vi "Pull_Data_via_Public_Client.vi"(0 "Path of File relative to EnFlo Data Root":path[](array[path]), 1 "application reference":refnum<vi>, 2 "Running on Server?":bool, 3 "Archive Files?":bool, 5 "error in (no error)":errorcluster) -> (6 "Error String":string, 7 "Problem Files":path[](array[path]), 8 "error out":errorcluster)   [LabVIEW 2018]
uses:
  Anemometry/Anemometry Sub Vis/Globals/Constants_global.vi
  Sub VIs/Harvest_Global.vi
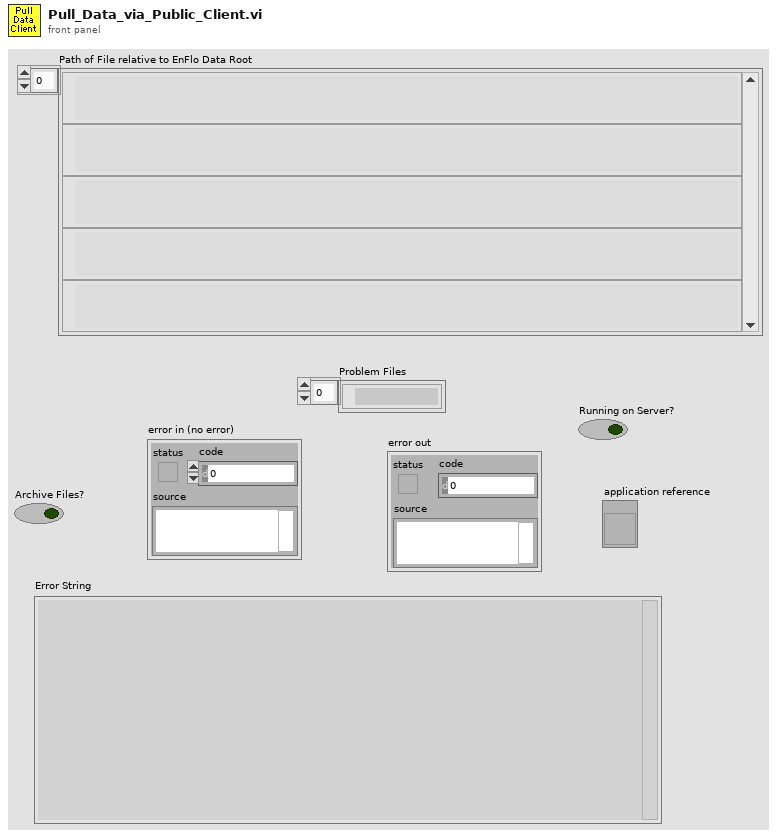
[diagram p1: front panel]
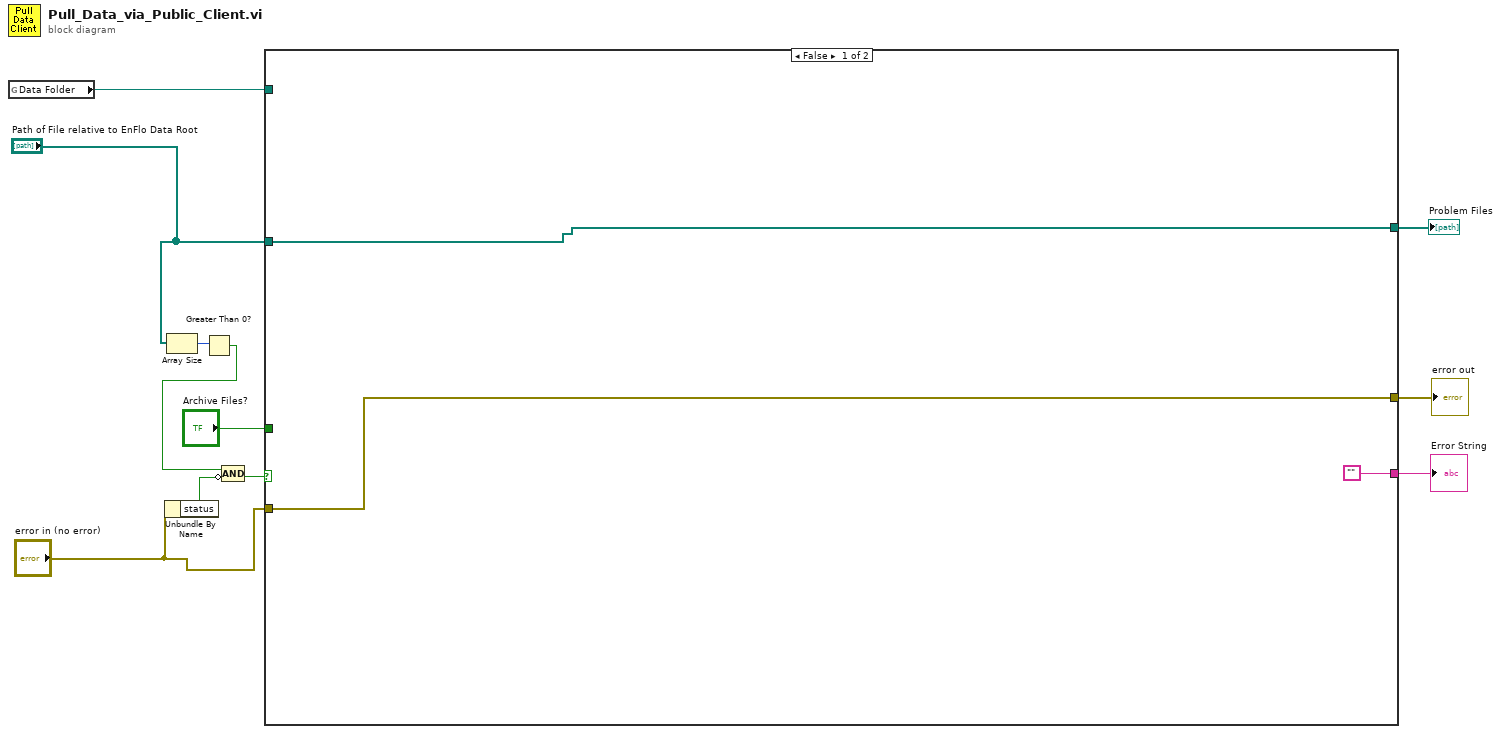
[diagram p0: block diagram]
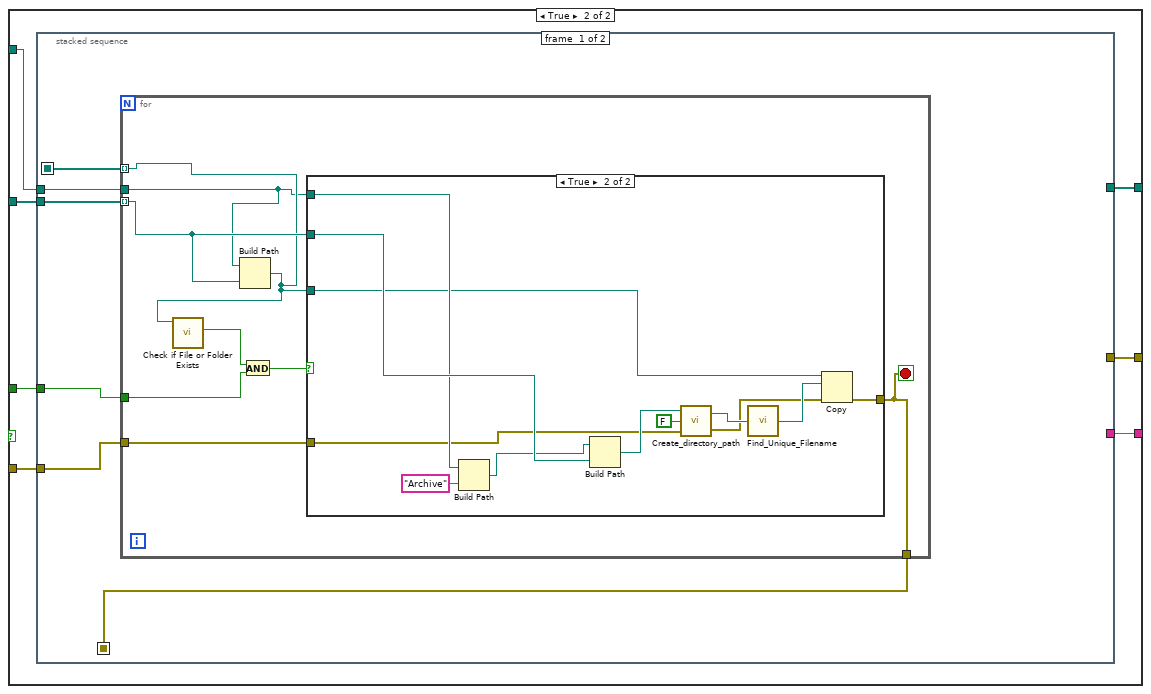
[diagram p2: hidden frame]
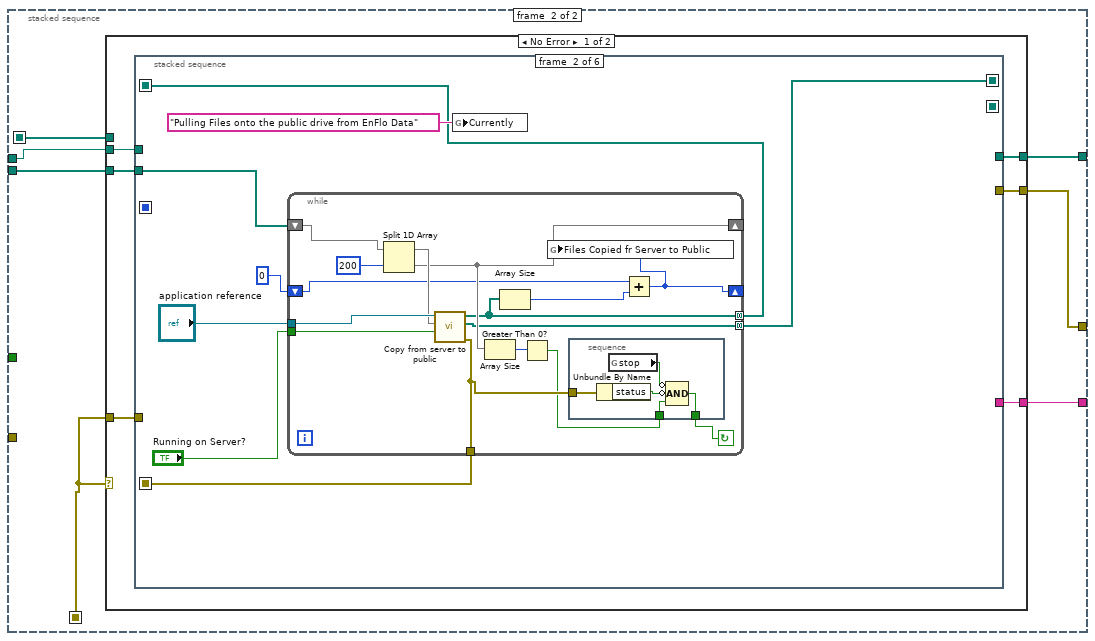
[diagram p4: hidden frame]
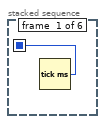
[diagram p5: hidden frame]
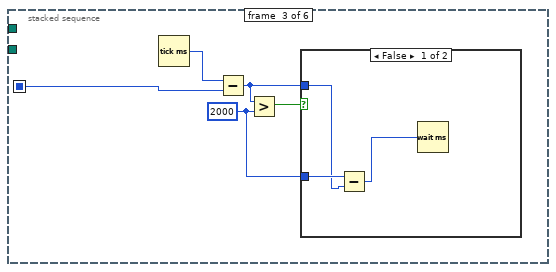
[diagram p6: hidden frame]
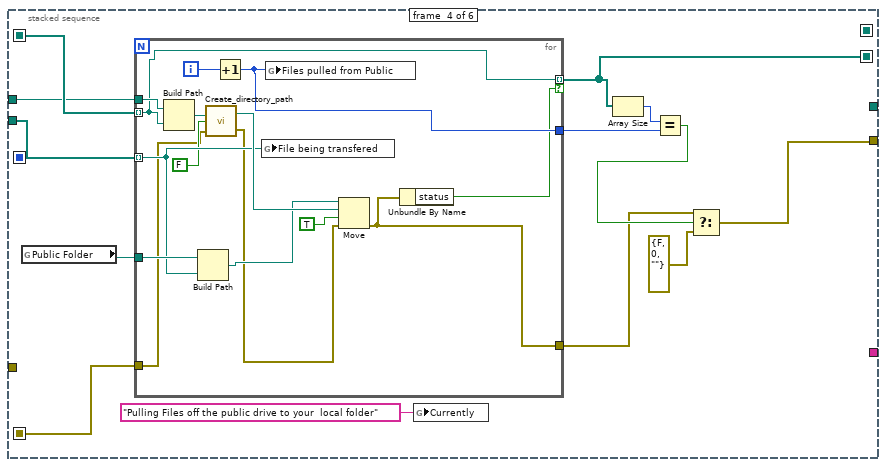
[diagram p8: hidden frame]
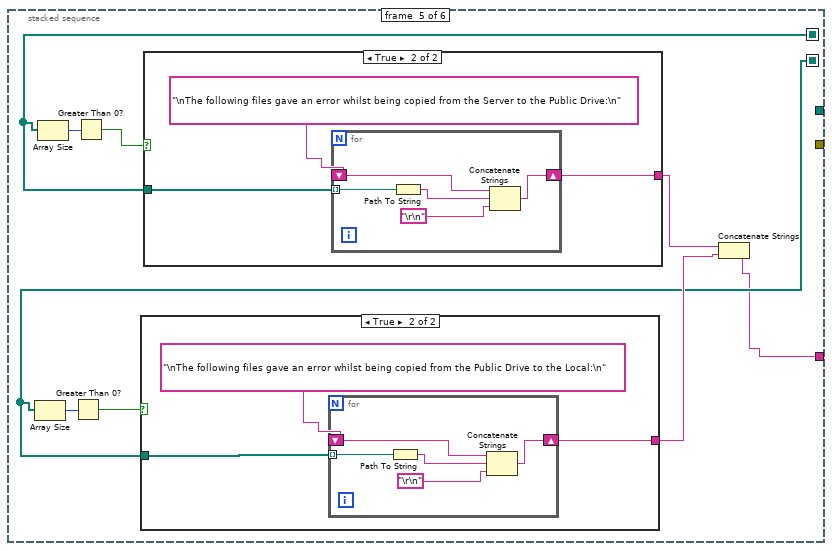
[diagram p9: hidden frame]
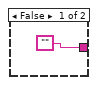
[diagram p10: hidden frame]
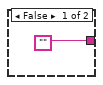
[diagram p11: hidden frame]
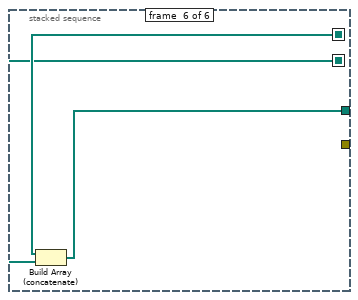
[diagram p12: hidden frame]
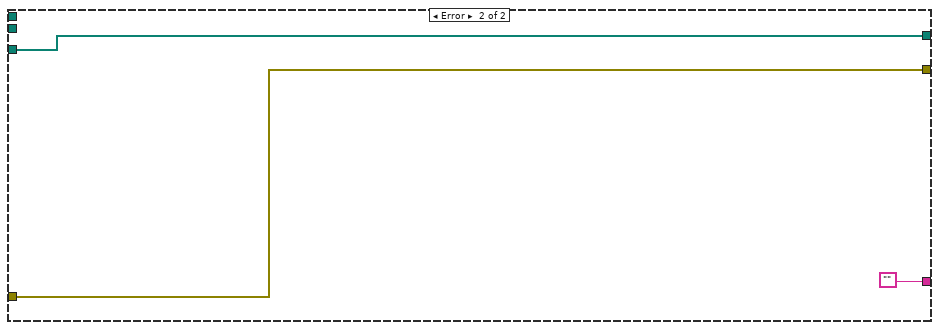
[diagram p13: hidden frame]
diagram:
  n1 = global read "Constants_global.vi" "Data Folder"() -> (w9:path)
  n2 = Unbundle By Name("error in (no error)") -> ("status"=w8:bool)
  n3 = Array Size(array="Path of File relative to EnFlo Data Root") -> (size(s)=w7:i32)
  n4 = Greater Than 0?(x=w7) -> (x > 0?=w6:bool)
  n5 = Compound Arithmetic op=AND(w6, invert w8) -> (w4:bool)
  n6 = case shown="False" w4 {
    tunnel: [w14 w21] -> w11
    tunnel: "error in (no error)" -> [w14 w20]
    tunnel: "Path of File relative to EnFlo Data Root" -> [w12 w19]
    tunnel: "Archive Files?" -> [_ w18]
    tunnel: w9 -> [_ w17]
    tunnel: ["" w16] -> w2
    tunnel: [w12 w15] -> w1
    frame False {
    }
    frame True {
      n7 = stacked-sequence {
        seq-local: [w26 _] -> [_ w52]
        seq-local: [w24 _] -> [_ w54]
        tunnel: [_ w55] -> w21
        tunnel: w20 -> [w27 _]
        tunnel: w19 -> [w25 w53]
        tunnel: w18 -> [w23 _]
        tunnel: w17 -> [w22 w51]
        tunnel: [_ w50] -> w16
        tunnel: [_ w49] -> w15
        frame #0 {
          n8 = for {
            tunnel: w27 -> [w35]
            tunnel: [w30] -> w26
            tunnel: w25 -> [w34] mode=indexing
            tunnel: w23 -> [w33]
            tunnel: [w29] -> w24 mode=indexing
            tunnel: w22 -> [w28]
            stop <- w30 stop-if-true
            n9 = Build Path(base path=w28, name or relative path=w34) -> (appended path=w29:path)
            n10 = call <vilib>:"Check if File or Folder Exists.vi"("path"=w29) -> ("file or folder exists?"=w32:bool)  [unwired: 8 in, 2 out]
            n11 = And(x=w32, y=w33) -> (x .and. y?=w31:bool)
            n12 = case shown="True" w31 {
              tunnel: w28 -> [_ w42]
              tunnel: w34 -> [_ w44]
              tunnel: [w36 w40] -> w30
              tunnel: w35 -> [w36 w39]
              tunnel: w29 -> [_ w38]
              frame False {
              }
              frame True {
                n13 = Build Path(base path=w42, name or relative path="Archive") -> (appended path=w41:path)
                n14 = Build Path(base path=w41, name or relative path=w44) -> (appended path=w47:path)
                n15 = call "Create_directory_path.vi"("error in (no error)"=w39, "Dialog Box"=FALSE, "Path name"=w47) -> ("error out"=w45:errorcluster, "Path name Out"=w46:path)
                n16 = call "Find_Unique_Filename.vi"("Path In"=w46) -> ("Unique Path Out"=w48:path)  [unwired: 2 in]
                n17 = Copy(8:w45, 10:w48, 11:w38) -> (0:w40:errorcluster)  [unwired: 2 in, 2 out]
              }
            }
          }
        }
        frame #1 {
          n18 = case shown="No Error" w52 {
            tunnel: [w59 w159] -> w55
            tunnel: w52 -> [w60 w159]
            tunnel: w54 -> [_ _]
            tunnel: w53 -> [w61 w157]
            tunnel: w51 -> [w58 _]
            tunnel: [w57 ""] -> w50
            tunnel: [w56 w157] -> w49
            frame No Error {
              n19 = stacked-sequence {
                seq-local: [_ w65 _ _ _ _] -> [_ _ _ w111 _ _]
                seq-local: [_ w69 _ _ _ _] -> [_ _ _ w108 _ _]
                seq-local: [w62 _ _ _ _ _] -> [_ _ w91 _ _ _]
                seq-local: [_ w63 _ _ _ _] -> [_ _ _ _ w129 w156]
                seq-local: [_ _ _ w99 _ _] -> [_ _ _ _ w128 w155]
                tunnel: w61 -> [_ w70 _ w109 _ _]
                tunnel: w60 -> [_ _ _ _ _ _]
                tunnel: [_ _ _ w100 _ _] -> w59
                tunnel: w58 -> [_ _ _ w107 _ _]
                tunnel: [_ _ _ _ w127 _] -> w57
                tunnel: [_ _ _ _ _ w154] -> w56
                frame #0 {
                  n20 = Tick Count (ms)() -> (millisecond timer value=w62:u32)
                }
                frame #1 {
                  n21 = while {
                    tunnel: [w80] -> w69
                    tunnel: "application reference" -> [w85]
                    tunnel: "Running on Server?" -> [w84]
                    shift-right: [w78] -> _
                    shift-left: w70 -> [w82]
                    tunnel: [w75] -> w65 mode=concatenating
                    shift-right: [w72] -> _
                    shift-left: 0 -> [w73]
                    tunnel: [w71] -> w63 mode=concatenating
                    stop <- w76 continue-if-true
                    n22 = Split 1D Array(array=w82, index=200) -> (first subarray=w81:path[], second subarray=w78:path[])
                    n23 = call "Copy from server to public.vi"("Running on Server?"=w84, "Path of File relative to EnFlo Data Root"=w81, "Application in"=w85) -> ("error out"=w80:errorcluster, "Problem Files"=w71:path[], "Relative Paths Out"=w75:path[])  [unwired: 6 in]
                    n24 = Array Size(array=w78) -> (size(s)=w79:i32)
                    n25 = Array Size(array=w75) -> (size(s)=w74:i32)
                    n26 = Greater Than 0?(x=w79) -> (x > 0?=w77:bool)
                    n27 = stacked-sequence {
                      tunnel: [w89] -> w76
                      tunnel: w80 -> [w87]
                      tunnel: w77 -> [w86]
                      frame #0 {
                        n28 = Unbundle By Name(w87) -> ("status"=w90:bool)
                        n29 = global read "Harvest_Global.vi" "stop"() -> (w88:bool)
                        n30 = Compound Arithmetic op=AND(invert w88, invert w90, w86) -> (w89:bool)
                      }
                    }
                    n31 = Add(x=w73, y=w74) -> (x+y=w72:i32)
                    n32 = global write "Harvest_Global.vi" "Files Copied fr Server to Public"(w72) -> ()
                  }
                  n33 = global write "Harvest_Global.vi" "Currently"("Pulling Files onto the public drive from EnFlo Data" ("Currently Running")) -> ()
                }
                frame #2 {
                  w94 = u32 2000 ("y")
                  n34 = Tick Count (ms)() -> (millisecond timer value=w92:u32)
                  n35 = Subtract(x=w92, y=w91) -> (x-y=w95:u32)
                  n36 = Greater?(x=w95, y=w94) -> (0:w93:bool)
                  n37 = case shown="False" w93 {
                    tunnel: w94 -> [w98 _]
                    tunnel: w95 -> [w97 _]
                    frame False {
                      n38 = Subtract(x=w98, y=w97) -> (x-y=w96:u32)
                      n39 = Wait (ms)(milliseconds to wait=w96) -> ()  [unwired: 1 out]
                    }
                    frame True {
                    }
                  }
                }
                frame #3 {
                  n40 = global read "Constants_global.vi" "Public Folder"() -> (w110:path)
                  n41 = for {
                    tunnel: w111 -> [w114] mode=indexing
                    tunnel: w110 -> [w125]
                    tunnel: w109 -> [w119] mode=indexing
                    tunnel: w108 -> [w117]
                    tunnel: [w123] -> w101
                    tunnel: w107 -> [w121]
                    tunnel: [w115] -> w104
                    tunnel: [w114] -> w99 mode=indexing if=w112
                    i -> [w120]
                    n42 = Build Path(base path=w121, name or relative path=w114) -> (appended path=w122:path)
                    n43 = Build Path(base path=w125, name or relative path=w119) -> (appended path=w124:path)
                    n44 = call "Create_directory_path.vi"("error in (no error)"=w117, "Dialog Box"=FALSE, "Path name"=w122) -> ("error out"=w116:errorcluster, "Path name Out"=w126:path)
                    n45 = Increment(x=w120) -> (x+1=w115:i32)
                    n46 = global write "Harvest_Global.vi" "File being transfered"(w119) -> ()
                    n47 = global write "Harvest_Global.vi" "Files pulled from Public"(w115) -> ()
                    n48 = Move(source path=w124, error in=w116, 9:TRUE ("overwrite (F)"), 10:w126) -> (error out=w123:errorcluster)  [unwired: 1 in, 2 out]
                    n49 = Unbundle By Name(w123) -> ("status"=w112:bool)
                  }
                  n50 = global write "Harvest_Global.vi" "Currently"("Pulling Files off the public drive to your  local folder" ("Currently Running")) -> ()
                  n51 = Array Size(array=w99) -> (size(s)=w105:i32)
                  n52 = Equal?(x=w105, y=w104) -> (x = y?=w102:bool)
                  n53 = Select(t=w101, s=w102, f=errorcluster {"status"=FALSE, "code"=0, "source"=""} ("error out")) -> (s? t:f=w100:errorcluster)
                }
                frame #4 {
                  n54 = Array Size(array=w128) -> (size(s)=w133:i32)
                  n55 = Array Size(array=w129) -> (size(s)=w130:i32)
                  n56 = Greater Than 0?(x=w133) -> (x > 0?=w132:bool)
                  n57 = Greater Than 0?(x=w130) -> (x > 0?=w131:bool)
                  n58 = case shown="True" w132 {
                    tunnel: w128 -> [_ w139]
                    tunnel: ["" w137] -> w135
                    frame False {
                    }
                    frame True {
                      n59 = for {
                        tunnel: w139 -> [w144] mode=indexing
                        shift-right: [w141] -> w137
                        shift-left: "\nThe following files gave an error whilst being copied from the Public Drive to the Local:\n" -> [w140]
                        n60 = Path To String(path=w144) -> (string=w143:string)
                        n61 = Concatenate Strings(w140, w143, "\r\n") -> (w141:string)
                      }
                    }
                  }
                  n62 = case shown="True" w131 {
                    tunnel: w129 -> [_ w148]
                    tunnel: ["" w146] -> w134
                    frame False {
                    }
                    frame True {
                      n63 = for {
                        tunnel: w148 -> [w153] mode=indexing
                        shift-right: [w150] -> w146
                        shift-left: "\nThe following files gave an error whilst being copied from the Server to the Public Drive:\n" -> [w149]
                        n64 = Path To String(path=w153) -> (string=w152:string)
                        n65 = Concatenate Strings(w149, w152, "\r\n") -> (w150:string)
                      }
                    }
                  }
                  n66 = Concatenate Strings(w134, w135) -> (w127:string)
                }
                frame #5 {
                  n67 = Build Array (concatenate)(w156, w155) -> (w154:path[])
                }
              }
            }
            frame Error {
            }
          }
        }
      }
    }
  }
  "error out" <- w11
  "Error String" <- w2
  "Problem Files" <- w1
